vi "Create.vi"(8 "error in (no error)":errorcluster) -> (0 "error out":errorcluster, 3 "Stop Pointer":refnum<class "Stop Pointer.lvclass">)   [LabVIEW 2020, in "Memory Manager.lvlib" / "Stop Pointer.lvclass"]
uses:
  Stop Pointer.lvclass
  C:/NetCore/niveristand-custom-device-development-tools/lv-memory-manager/Source/Classes/Pointer/Pointer.lvclass
  Pointer.lvclass
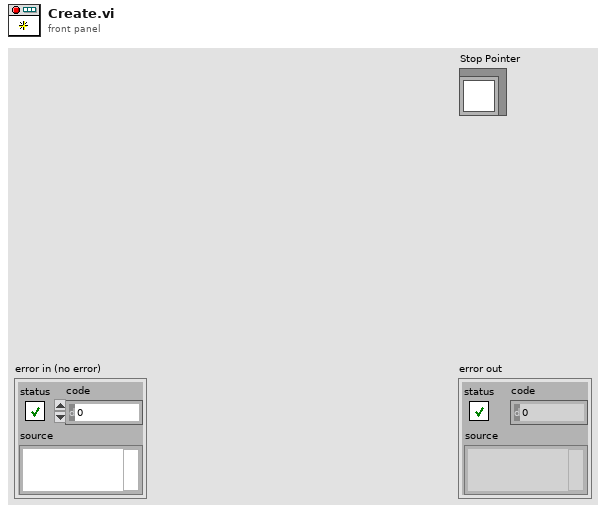
[diagram p1: front panel]
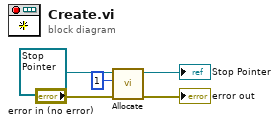
[diagram p0: block diagram]
diagram:
  n1 = call "Allocate.vi"("error in (no error)"="error in (no error)", "size"=u64 1, "Pointer type"=refnum<class "Stop Pointer.lvclass"> refnum ("Stop Pointer in")) -> ("error out"=→"error out":errorcluster, "Pointer out"=→"Stop Pointer":refnum<class "Stop Pointer.lvclass">)  [unwired: 7 in]
